vi "Jacobian_stuff.vi"(6 "Linear velocities":dbl[](array[numeric]), 7 "Timestep":dbl=0.1, 8 "L2":dbl=30.0, 9 "L1":dbl=30.0, 10 "Angles (degrees)":dbl[](array[numeric])=[30.0, 120.0], 11 "Loops":i32=5) -> (2 "RPM Output":cluster{dbl, dbl}[](array[cluster]), 3 "2D Picture":picture)   [LabVIEW 2024]
uses:
  <vilib>/Analysis/baseanly.llb/Real Inverse Matrix.vi
  <vilib>/Analysis/baseanly.llb/A x Vector.vi
  <vilib>/Analysis/NI_AALBase.lvlib
panel:
  out "Bundled Angle Output":cluster{dbl, dbl}[](array[cluster])
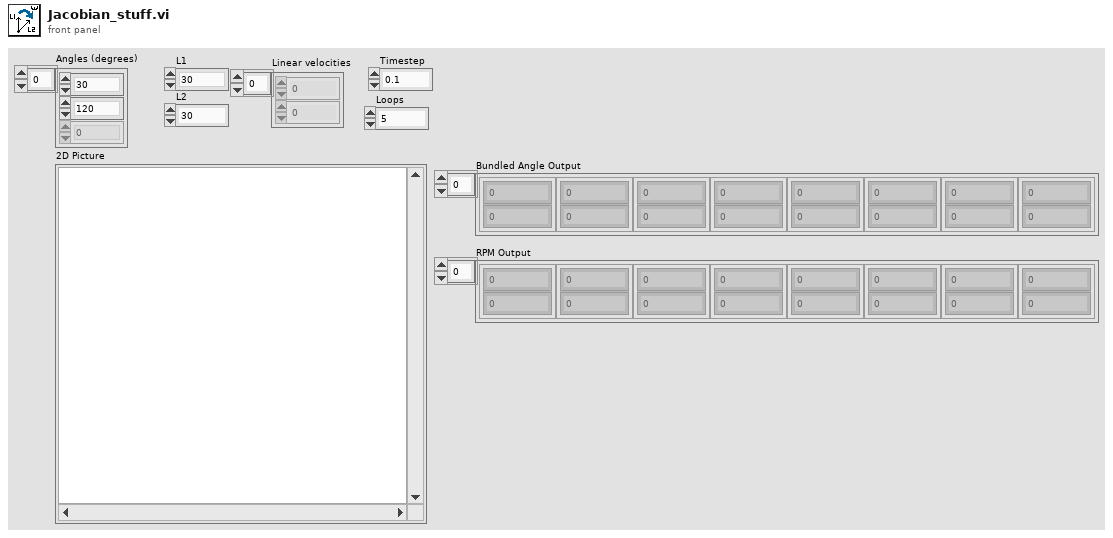
[diagram p1: front panel]
types:
  T1 = cluster{"L1":dbl, "L2":dbl, "Angles (degrees)":dbl[]}
  T2 = typedef "NI_Matrix.lvlib/RealMatrix.ctl" = dbl[][]
  T3 = cluster{"A x Vector[0]":dbl, "A x Vector[1]":dbl}
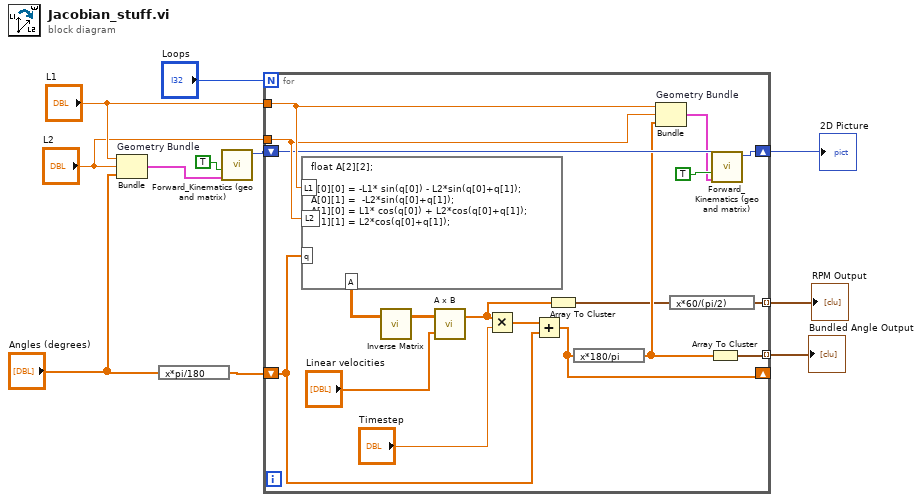
[diagram p0: block diagram]
diagram:
  n1 = Bundle "Geometry Bundle"("L1"="L1", "L2"="L2", "Angles (degrees)"="Angles (degrees)") -> (w9:T1)  [unwired: 1 in]
  n2 = expression code="x*pi/180"("Angles (degrees)") -> (w6:dbl[])
  n3 = call "Forward_Kinematics (geo and matrix).vi"("geometry"=w9, "geometry?"=TRUE) -> ("2D Picture"=w7:picture)  [unwired: 7 in, 2 out]
  n4 = for {
    N: "Loops" -> [_]
    tunnel: "L1" -> [w24]
    tunnel: "L2" -> [w23]
    shift-right: [w18] -> _
    shift-left: w6 -> [w20]
    shift-right: [w17] -> w4
    shift-left: w7 -> [w22]
    tunnel: [w15] -> w2 mode=indexing
    tunnel: [w12] -> w1 mode=indexing
    n5 = formula code="float A[2][2];\n\nA[0][0] = -L1* sin(q[0]) - L2*sin(q[0]+q[1]);\nA[0][1] =  -L2*sin(q[0]+q[1]);\nA[1][0] = L1* cos(q[0]) + L2*cos(q[0]+q[1]);\nA[1][1] = L2*cos(q[0]+q[1]);"("q"=w20, "L1"=w24, "L2"=w23) -> ("A"=w29:dbl[][])
    n6 = call-poly <vilib>:"Inverse Matrix.vi"("Input Matrix"=w29) -> ("Inverse Matrix"=w28:T2)  [unwired: 1 in, 1 out]
    n7 = call-poly <vilib>:"A x B.vi"("Vector"="Linear velocities", "A"=w28) -> ("A x Vector"=w14:dbl[])  [unwired: 1 out]
    n8 = Multiply(x=w14, y="Timestep") -> (x*y=w21:dbl[])
    n9 = Add(x=w21, y=w20) -> (x+y=w18:dbl[])
    n10 = Array To Cluster(array=w14) -> (cluster=w13:T3)
    n11 = expression code="x*180/pi"(w18) -> (w16:dbl[])
    n12 = Bundle "Geometry Bundle"("L1"=w24, "L2"=w23, w16) -> (w19:cluster{"L1":dbl, "L2":dbl, dbl[]})  [unwired: 1 in]
    n13 = expression code="x*60/(pi/2)"(w13) -> (w12:T3)
    n14 = Array To Cluster(array=w16) -> (cluster=w15:cluster{"[0]":dbl, "[1]":dbl})
    n15 = call "Forward_Kinematics (geo and matrix).vi"("geometry"=w19, "geometry?"=TRUE, "picture in"=w22) -> ("2D Picture"=w17:picture)  [unwired: 6 in, 2 out]
  }
  "2D Picture" <- w4
  "Bundled Angle Output" <- w2
  "RPM Output" <- w1
